vi "MNIST_Classifier_CNN(Train).vi"() -> ()   [LabVIEW 2024]
doc: "This example demonstrates the usage of Deep Learning Toolkit for solving hand written digit recognition problem with Convolutional Neural Network (CNN).\n\nDataset: MNIST http://yann.lecun.com/exdb/mnist/\nRequirements: Deep Learning Toolkit for LabVIEW."
uses:
  <vilib>/Ngene/Deep Learning Toolkit/Toolkit/NN_Train/Controls/NN_Train_Params.ctl
  <vilib>/Ngene/Deep Learning Toolkit/Toolkit/NN_Train/Controls/NN_Train_Optimizer.ctl
  <vilib>/Ngene/Deep Learning Toolkit/Toolkit/NN_Train/Controls/NN_Train_Data_Sampling.ctl
  _Controls/Img_GrayScale.ctl
  <vilib>/Ngene/Deep Learning Toolkit/Toolkit/NN_Train/Controls/NN_Train_Session_Data.ctl
  <vilib>/Ngene/Deep Learning Toolkit/Toolkit/NN_Train/Controls/NN_LR_Policy_Cfg.ctl
  <vilib>/Ngene/Deep Learning Toolkit/Toolkit/NN_Train/Controls/NN_LR_Policy_Type.ctl
  <vilib>/Ngene/Deep Learning Toolkit/Toolkit/NN_Network/Controls/NN_Device.ctl
  <vilib>/Ngene/Deep Learning Toolkit/Toolkit/NN_Layers/Layers/Conv2D/Controls/NN_Layer_Config(Conv2D).ctl
  <vilib>/Ngene/Deep Learning Toolkit/Toolkit/NN_Layers/Layers/Conv2D/Controls/NN_Layer_Params(Conv2D).ctl
  <vilib>/Ngene/Deep Learning Toolkit/Toolkit/NN_Layers/Layers/Conv2D/Controls/NN_Conv2D_Padding_Type.ctl
  <vilib>/Ngene/Deep Learning Toolkit/Toolkit/NN_Layers/Layers/BatchNorm/Controls/NN_BN_Params.ctl
  <vilib>/Ngene/Deep Learning Toolkit/Toolkit/NN_Activations/Controls/NN_Activation_Type.ctl
  <vilib>/Ngene/Deep Learning Toolkit/Toolkit/NN_Layers/Controls/NN_Layer_Init_Params.ctl
  <vilib>/Ngene/Deep Learning Toolkit/Toolkit/NN_Layers/Controls/NN_Layer_Weight_Init_Type.ctl
  <vilib>/Ngene/Deep Learning Toolkit/Toolkit/NN_Layers/Layers/FC/Controls/NN_Layer_Config(FC).ctl
  <vilib>/Ngene/Deep Learning Toolkit/Toolkit/NN_Network/Controls/NN_Save_Before_Destroy_Options.ctl
  <vilib>/Ngene/Deep Learning Toolkit/Toolkit/NN_Layers/Layers/Input/Controls/NN_Layer_Config(Input3D).ctl
  <vilib>/Ngene/Deep Learning Toolkit/Toolkit/NN_Data/API/NN_Dims(C,H,W).ctl
  <vilib>/Ngene/Deep Learning Toolkit/Toolkit/NN_Data/Controls/NN_Data_type.ctl
  <vilib>/Ngene/Deep Learning Toolkit/Toolkit/NN_Layers/Layers/Input/NN_Layer_Create(Input3D).vi
  <vilib>/Ngene/Deep Learning Toolkit/Toolkit/NN_Layers/Layers/Conv2D/NN_Layer_Create(Conv2D).vi
  <vilib>/Ngene/Deep Learning Toolkit/Toolkit/NN_Layers/Layers/FC/NN_Layer_Create(FC).vi
  <vilib>/Ngene/Deep Learning Toolkit/Toolkit/NN_Layers/Layers/SoftMax/NN_Layer_Create(SoftMax).vi
  <vilib>/Ngene/Deep Learning Toolkit/Toolkit/NN_Train/Loss_Functions/NN_Set_Loss(CrossEntropy).vi
  <vilib>/ptbypt/Filters.llb/FIR Filter PtByPt.vi
  <vilib>/Ngene/Deep Learning Toolkit/Toolkit/NN_Network/subVIs/NN_Predict/NN_Predict(In3D_Out1D).vi
  <vilib>/Ngene/Deep Learning Toolkit/Toolkit/NN_Train/Eval_Loss/NN_Eval_Test_Error_Loss/NN_Eval(In3D_Out1D).vi
  <vilib>/Ngene/Deep Learning Toolkit/Toolkit/NN_Train/Eval_Loss/NN_Calc_Cofusion_Matrix/NN_Calc_Confusion_Matrix(In3D_Out1D).vi
  <vilib>/Ngene/Deep Learning Toolkit/Toolkit/NN_Data/subVIs/Dataset_Destroy/NN_Datasets_All_Destroy(In3D_Out1D).vi
  <vilib>/Ngene/Deep Learning Toolkit/Toolkit/NN_Network/API/NN_Set_Input/3D/NN_Set_Input(3D_SGL_idx).vi
  <vilib>/Ngene/Deep Learning Toolkit/Toolkit/Deep_Learning_Toolkit_by_Ngene.lvlib
panel:
  in  "Tab":T1(tab)
  out "Train Speed (img/s)":dbl=1568.329544559763 format="%#_3p"
  out "Train Graphs":T2(graph)
  in  "Check_Vald":bool
  out "Session Data":T3={"Epochs"=0.22905263, "Tot_Iter"=102, "LR"=0.02, "LR_iter"=103}
  in  "Stop_Train":bool
  out "Train/Val_Metrics":T4={"Train_Loss"=0.05827807, "Valid_Loss"=0.04526825, "Valid_Error"=0.042666666} {"Train_Loss" format="%#_4g"; "Valid_Loss" format="%#_3g"}
  in  "LR Update Policy":T5={"Policy_Type"=enum."Step", "LR0"=0.019999999998737077, "k"=4.0, "WarmUp_Policy"=enum."Step", "WarmUp_Iter"=1, "WarmUp_Ratio"=1.0} {"WarmUp_Ratio" min=1; "WarmUp_Iter" min=1; "LR0" format="%.7f"}
  out "Train Speed (s/iter)":dbl=0.08161550003569573 format="%#_2p"
  in  "Train_Params":T7={"Optimizer"=enum."SGD", "Beta_1"=0.9, "Beta_2"=0.999, "Weight Decay(L1)"=1e-07, "Weight Decay(L2)"=1e-07, "Data_Sampling"=enum."Random"}
  out "Time_Elapsed":dbl=8.652226000092924 format="%<%H:%M:%S>t"
  out "Test_Loss":sgl=0.046575993 format="%#_3g"
  out "Test_Error":sgl=0.044
  in  "Working Dir":path=path "D:/working"
  in  "MNIST Dataset Path":path
  in  "NN_Device":T10
  out "Labels":string[](array[string])=["0", "1", "2", "3", "4", "5", "6", "7", "8", "9"]
  out "Draw Digit (280x280 px)":picture
  in  "Pen Color":u32(colorbox)=197379
  in  "Clear":bool
  out "Test Speed (img/s)":dbl=119.97888344398501 format="%#_2p"
  out "test time(s/img)":dbl=0.008334800018928945 format="%#_3p"
  out "Predictions":sgl[](array[slide])=[0.00022317072, 0.0016224136, 0.00590554, 0.9895844, 0.0010204009, 0.00023260966, 0.00083900435, 0.00020435848, 0.00020539068, 0.00016265694] scale=0.0..1.0
  in  "Pen Width":dbl=24.0
  in  "Stop Test":bool
  out "Pen Attributes":T11={"Width"=26, "Style"=enum."Solid"}
  out "image (28x28px)":sgl[][](graph)=[[-1.0, -1.0, -1.0, -1.0, -1.0, -1.0, -1.0, -1.0, -1.0, -1.0, -1.0, -1.0, -1.0, -1.0, -1.0, -1.0, -1.0, -1.0, -1.0, -1.0, -1.0, -1.0, -1.0, -1.0, -1.0, -1.0, -1.0, -1.0], [-1.0, -1.0, -1.0, -1.0, -1.0, -1.0, -1.0, -1.0, -1.0, -1.0, -1.0, -1.0, -1.0, -1.0, -1.0, -1.0, -1.0, -1.0, -1.0, -1.0, -1.0, -1.0, -1.0, -1.0, -1.0, -1.0, -1.0, -1.0], [-1.0, -1.0, -1.0, -1.0, -1.0, -1.0, -1.0, -1.0, -1.0, -1.0, -1.0, -1.0, -1.0, -1.0, -1.0, -1.0, -1.0, -1.0, -1.0, -1.0, -1.0, -1.0, -1.0, -1.0, -1.0, -1.0, -1.0, -1.0], [-1.0, -1.0, -1.0, -1.0, -1.0, -1.0, -1.0, -1.0, -1.0, -1.0, -1.0, -1.0, -1.0, -1.0, -1.0, -1.0, -1.0, -1.0, -1.0, -1.0, -1.0, -1.0, -1.0, -1.0, -1.0, -1.0, -1.0, -1.0], [-1.0, -1.0, -1.0, -1.0, -1.0, -1.0, -1.0, -1.0, -1.0, -1.0, -1.0, -1.0, -1.0, -1.0, -1.0, -1.0, -1.0, -1.0, -1.0, -1.0, -1.0, -1.0, -1.0, -1.0, -1.0, -1.0, -1.0, -1.0], [-1.0, -1.0, -1.0, -1.0, -1.0, -1.0, -1.0, -1.0, -1.0, -1.0, -1.0, -1.0, -1.0, -1.0, -1.0, -1.0, -1.0, -1.0, -1.0, -1.0, -1.0, -1.0, -1.0, -1.0, -1.0, -1.0, -1.0, -1.0], [-1.0, -1.0, -1.0, -1.0, -1.0, -1.0, -1.0, -1.0, -1.0, -1.0, -1.0, -1.0, -1.0, -1.0, -1.0, -1.0, -1.0, -1.0, -1.0, -1.0, -1.0, -1.0, -1.0, -1.0, -1.0, -1.0, -1.0, -1.0], [-1.0, -1.0, -1.0, -1.0, -1.0, -1.0, -1.0, -1.0, -1.0, -1.0, -1.0, -1.0, -1.0, -1.0, -1.0, -1.0, -1.0, -1.0, -1.0, -1.0, -1.0, -1.0, -1.0, -1.0, -1.0, -1.0, -1.0, -1.0], [-1.0, -1.0, -1.0, -1.0, -1.0, -1.0, -1.0, -1.0, -1.0, -1.0, -1.0, -1.0, -1.0, -1.0, -1.0, -1.0, -1.0, -1.0, -1.0, -1.0, -1.0, -1.0, -1.0, -1.0, -1.0, -1.0, -1.0, -1.0], [-1.0, -1.0, -1.0, -1.0, -1.0, -1.0, -1.0, -1.0, -1.0, -1.0, -1.0, -1.0, -1.0, -1.0, -1.0, -1.0, -1.0, -1.0, -1.0, -1.0, -1.0, -1.0, -1.0, -1.0, -1.0, -1.0, -1.0, -1.0], [-1.0, -1.0, -1.0, -1.0, -1.0, -1.0, -1.0, -1.0, -1.0, -1.0, -1.0, -1.0, -1.0, -1.0, -1.0, -1.0, -1.0, -1.0, -1.0, -1.0, -1.0, -1.0, -1.0, -1.0, -1.0, -1.0, -1.0, -1.0], [-1.0, -1.0, -1.0, -1.0, -1.0, -1.0, -1.0, -1.0, -1.0, -1.0, -1.0, -1.0, -1.0, -1.0, -1.0, -1.0, -1.0, -1.0, -1.0, -1.0, -1.0, -1.0, -1.0, -1.0, -1.0, -1.0, -1.0, -1.0], [-1.0, -1.0, -1.0, -1.0, -1.0, -1.0, -1.0, -1.0, -1.0, -1.0, -1.0, -1.0, -1.0, -1.0, -1.0, -1.0, -1.0, -1.0, -1.0, -1.0, -1.0, -1.0, -1.0, -1.0, -1.0, -1.0, -1.0, -1.0], [-1.0, -1.0, -1.0, -1.0, -1.0, -1.0, -1.0, -1.0, -1.0, -1.0, -1.0, -1.0, -1.0, -1.0, -1.0, -1.0, -1.0, -1.0, -1.0, -1.0, -1.0, -1.0, -1.0, -1.0, -1.0, -1.0, -1.0, -1.0], [-1.0, -1.0, -1.0, -1.0, -1.0, -1.0, -1.0, -1.0, -1.0, -1.0, -1.0, -1.0, -1.0, -1.0, -1.0, -1.0, -1.0, -1.0, -1.0, -1.0, -1.0, -1.0, -1.0, -1.0, -1.0, -1.0, -1.0, -1.0], [-1.0, -1.0, -1.0, -1.0, -1.0, -1.0, -1.0, -1.0, -1.0, -1.0, -1.0, -1.0, -1.0, -1.0, -1.0, -1.0, -1.0, -1.0, -1.0, -1.0, -1.0, -1.0, -1.0, -1.0, -1.0, -1.0, -1.0, -1.0], [-1.0, -1.0, -1.0, -1.0, -1.0, -1.0, -1.0, -1.0, -1.0, -1.0, -1.0, -1.0, -1.0, -1.0, -1.0, -1.0, -1.0, -1.0, -1.0, -1.0, -1.0, -1.0, -1.0, -1.0, -1.0, -1.0, -1.0, -1.0], [-1.0, -1.0, -1.0, -1.0, -1.0, -1.0, -1.0, -1.0, -1.0, -1.0, -1.0, -1.0, -1.0, -1.0, -1.0, -1.0, -1.0, -1.0, -1.0, -1.0, -1.0, -1.0, -1.0, -1.0, -1.0, -1.0, -1.0, -1.0], [-1.0, -1.0, -1.0, -1.0, -1.0, -1.0, -1.0, -1.0, -1.0, -1.0, -1.0, -1.0, -1.0, -1.0, -1.0, -1.0, -1.0, -1.0, -1.0, -1.0, -1.0, -1.0, -1.0, -1.0, -1.0, -1.0, -1.0, -1.0], [-1.0, -1.0, -1.0, -1.0, -1.0, -1.0, -1.0, -1.0, -1.0, -1.0, -1.0, -1.0, -1.0, -1.0, -1.0, -1.0, -1.0, -1.0, -1.0, -1.0, -1.0, -1.0, -1.0, -1.0, -1.0, -1.0, -1.0, -1.0], [-1.0, -1.0, -1.0, -1.0, -1.0, -1.0, -1.0, -1.0, -1.0, -1.0, -1.0, -1.0, -1.0, -1.0, -1.0, -1.0, -1.0, -1.0, -1.0, -1.0, -1.0, -1.0, -1.0, -1.0, -1.0, -1.0, -1.0, -1.0], [-1.0, -1.0, -1.0, -1.0, -1.0, -1.0, -1.0, -1.0, -1.0, -1.0, -1.0, -1.0, -1.0, -1.0, -1.0, -1.0, -1.0, -1.0, -1.0, -1.0, -1.0, -1.0, -1.0, -1.0, -1.0, -1.0, -1.0, -1.0], [-1.0, -1.0, -1.0, -1.0, -1.0, -1.0, -1.0, -1.0, -1.0, -1.0, -1.0, -1.0, -1.0, -1.0, -1.0, -1.0, -1.0, -1.0, -1.0, -1.0, -1.0, -1.0, -1.0, -1.0, -1.0, -1.0, -1.0, -1.0], [-1.0, -1.0, -1.0, -1.0, -1.0, -1.0, -1.0, -1.0, -1.0, -1.0, -1.0, -1.0, -1.0, -1.0, -1.0, -1.0, -1.0, -1.0, -1.0, -1.0, -1.0, -1.0, -1.0, -1.0, -1.0, -1.0, -1.0, -1.0], [-1.0, -1.0, -1.0, -1.0, -1.0, -1.0, -1.0, -1.0, -1.0, -1.0, -1.0, -1.0, -1.0, -1.0, -1.0, -1.0, -1.0, -1.0, -1.0, -1.0, -1.0, -1.0, -1.0, -1.0, -1.0, -1.0, -1.0, -1.0], [-1.0, -1.0, -1.0, -1.0, -1.0, -1.0, -1.0, -1.0, -1.0, -1.0, -1.0, -1.0, -1.0, -1.0, -1.0, -1.0, -1.0, -1.0, -1.0, -1.0, -1.0, -1.0, -1.0, -1.0, -1.0, -1.0, -1.0, -1.0], [-1.0, -1.0, -1.0, -1.0, -1.0, -1.0, -1.0, -1.0, -1.0, -1.0, -1.0, -1.0, -1.0, -1.0, -1.0, -1.0, -1.0, -1.0, -1.0, -1.0, -1.0, -1.0, -1.0, -1.0, -1.0, -1.0, -1.0, -1.0], [-1.0, -1.0, -1.0, -1.0, -1.0, -1.0, -1.0, -1.0, -1.0, -1.0, -1.0, -1.0, -1.0, -1.0, -1.0, -1.0, -1.0, -1.0, -1.0, -1.0, -1.0, -1.0, -1.0, -1.0, -1.0, -1.0, -1.0, -1.0]]
  out "Incorrectly Classified Imgs":T12[][](array[typedef])=[[{"image"=array28x28[784 elements], "Truth"=2, "Predicted"=2}, {"image"=array28x28[784 elements], "Truth"=9, "Predicted"=9}, {"image"=array28x28[784 elements], "Truth"=2, "Predicted"=2}, {"image"=array28x28[784 elements], "Truth"=7, "Predicted"=7}, {"image"=array28x28[784 elements], "Truth"=8, "Predicted"=8}, {"image"=array28x28[784 elements], "Truth"=2, "Predicted"=2}, {"image"=array28x28[784 elements], "Truth"=0, "Predicted"=0}, {"image"=array28x28[784 elements], "Truth"=1, "Predicted"=1}, {"image"=array28x28[784 elements], "Truth"=7, "Predicted"=7}, {"image"=array28x28[784 elements], "Truth"=3, "Predicted"=3}], [{"image"=array28x28[784 elements], "Truth"=7, "Predicted"=7}, {"image"=array28x28[784 elements], "Truth"=7, "Predicted"=7}, {"image"=array28x28[784 elements], "Truth"=7, "Predicted"=7}, {"image"=array28x28[784 elements], "Truth"=7, "Predicted"=7}, {"image"=array28x28[784 elements], "Truth"=0, "Predicted"=0}, {"image"=array28x28[784 elements], "Truth"=5, "Predicted"=5}, {"image"=array28x28[784 elements], "Truth"=2, "Predicted"=2}, {"image"=array28x28[784 elements], "Truth"=5, "Predicted"=5}, {"image"=array28x28[784 elements], "Truth"=8, "Predicted"=8}, {"image"=array28x28[784 elements], "Truth"=5, "Predicted"=5}], [{"image"=array28x28[784 elements], "Truth"=1, "Predicted"=1}, {"image"=array28x28[784 elements], "Truth"=9, "Predicted"=9}, {"image"=array28x28[784 elements], "Truth"=7, "Predicted"=7}, {"image"=array28x28[784 elements], "Truth"=2, "Predicted"=2}, {"image"=array28x28[784 elements], "Truth"=3, "Predicted"=3}, {"image"=array28x28[784 elements], "Truth"=9, "Predicted"=9}, {"image"=array28x28[784 elements], "Truth"=2, "Predicted"=2}, {"image"=array28x28[784 elements], "Truth"=7, "Predicted"=7}, {"image"=array28x28[784 elements], "Truth"=8, "Predicted"=8}, {"image"=array28x28[784 elements], "Truth"=4, "Predicted"=4}], [{"image"=array28x28[784 elements], "Truth"=0, "Predicted"=0}, {"image"=array28x28[784 elements], "Truth"=8, "Predicted"=8}, {"image"=array28x28[784 elements], "Truth"=3, "Predicted"=3}, {"image"=array28x28[784 elements], "Truth"=4, "Predicted"=4}, {"image"=array28x28[784 elements], "Truth"=9, "Predicted"=9}, {"image"=array28x28[784 elements], "Truth"=6, "Predicted"=6}, {"image"=array28x28[784 elements], "Truth"=9, "Predicted"=9}, {"image"=array28x28[784 elements], "Truth"=9, "Predicted"=9}, {"image"=array28x28[784 elements], "Truth"=5, "Predicted"=5}, {"image"=array28x28[784 elements], "Truth"=9, "Predicted"=9}], [{"image"=array28x28[784 elements], "Truth"=3, "Predicted"=3}, {"image"=array28x28[784 elements], "Truth"=7, "Predicted"=7}, {"image"=array28x28[784 elements], "Truth"=9, "Predicted"=9}, {"image"=array28x28[784 elements], "Truth"=7, "Predicted"=7}, {"image"=array28x28[784 elements], "Truth"=3, "Predicted"=3}, {"image"=array28x28[784 elements], "Truth"=7, "Predicted"=7}, {"image"=array28x28[784 elements], "Truth"=5, "Predicted"=5}, {"image"=array28x28[784 elements], "Truth"=7, "Predicted"=7}, {"image"=array28x28[784 elements], "Truth"=6, "Predicted"=6}, {"image"=array28x28[784 elements], "Truth"=9, "Predicted"=9}], [{"image"=array28x28[784 elements], "Truth"=0, "Predicted"=0}, {"image"=array28x28[784 elements], "Truth"=9, "Predicted"=9}, {"image"=array28x28[784 elements], "Truth"=2, "Predicted"=2}, {"image"=array28x28[784 elements], "Truth"=9, "Predicted"=9}, {"image"=array28x28[784 elements], "Truth"=5, "Predicted"=5}, {"image"=array28x28[784 elements], "Truth"=1, "Predicted"=1}, {"image"=array28x28[784 elements], "Truth"=8, "Predicted"=8}, {"image"=array28x28[784 elements], "Truth"=7, "Predicted"=7}, {"image"=array28x28[784 elements], "Truth"=4, "Predicted"=4}, {"image"=array28x28[784 elements], "Truth"=0, "Predicted"=0}], [{"image"=array28x28[784 elements], "Truth"=8, "Predicted"=8}, {"image"=array28x28[784 elements], "Truth"=6, "Predicted"=6}, {"image"=array28x28[784 elements], "Truth"=8, "Predicted"=8}, {"image"=array28x28[784 elements], "Truth"=1, "Predicted"=1}, {"image"=array28x28[784 elements], "Truth"=7, "Predicted"=7}, {"image"=array28x28[784 elements], "Truth"=7, "Predicted"=7}, {"image"=array28x28[784 elements], "Truth"=7, "Predicted"=7}, {"image"=array28x28[784 elements], "Truth"=2, "Predicted"=2}, {"image"=array28x28[784 elements], "Truth"=2, "Predicted"=2}, {"image"=array28x28[784 elements], "Truth"=4, "Predicted"=4}], [{"image"=array28x28[784 elements], "Truth"=5, "Predicted"=5}, {"image"=array28x28[784 elements], "Truth"=6, "Predicted"=6}, {"image"=array28x28[784 elements], "Truth"=1, "Predicted"=1}, {"image"=array28x28[784 elements], "Truth"=9, "Predicted"=9}, {"image"=array28x28[784 elements], "Truth"=9, "Predicted"=9}, {"image"=array28x28[784 elements], "Truth"=7, "Predicted"=7}, {"image"=array28x28[784 elements], "Truth"=3, "Predicted"=3}, {"image"=array28x28[784 elements], "Truth"=2, "Predicted"=2}, {"image"=array28x28[784 elements], "Truth"=6, "Predicted"=6}, {"image"=array28x28[784 elements], "Truth"=3, "Predicted"=3}], [{"image"=array28x28[784 elements], "Truth"=9, "Predicted"=9}, {"image"=array28x28[784 elements], "Truth"=5, "Predicted"=5}, {"image"=array28x28[784 elements], "Truth"=1, "Predicted"=1}, {"image"=array28x28[784 elements], "Truth"=0, "Predicted"=0}, {"image"=array28x28[784 elements], "Truth"=5, "Predicted"=5}, {"image"=array28x28[784 elements], "Truth"=7, "Predicted"=7}, {"image"=array28x28[784 elements], "Truth"=2, "Predicted"=2}, {"image"=array28x28[784 elements], "Truth"=5, "Predicted"=5}, {"image"=array28x28[784 elements], "Truth"=7, "Predicted"=7}, {"image"=array28x28[784 elements], "Truth"=4, "Predicted"=4}], [{"image"=array28x28[784 elements], "Truth"=9, "Predicted"=9}, {"image"=array28x28[784 elements], "Truth"=9, "Predicted"=9}, {"image"=array28x28[784 elements], "Truth"=5, "Predicted"=5}, {"image"=array28x28[784 elements], "Truth"=5, "Predicted"=5}, {"image"=array28x28[784 elements], "Truth"=3, "Predicted"=3}, {"image"=array28x28[784 elements], "Truth"=6, "Predicted"=6}, {"image"=array28x28[784 elements], "Truth"=7, "Predicted"=7}, {"image"=array28x28[784 elements], "Truth"=7, "Predicted"=7}, {"image"=array28x28[784 elements], "Truth"=7, "Predicted"=7}, {"image"=array28x28[784 elements], "Truth"=3, "Predicted"=3}], [{"image"=array28x28[784 elements], "Truth"=3, "Predicted"=3}, {"image"=array28x28[784 elements], "Truth"=7, "Predicted"=7}, {"image"=array28x28[784 elements], "Truth"=5, "Predicted"=5}, {"image"=array28x28[784 elements], "Truth"=3, "Predicted"=3}, {"image"=array28x28[784 elements], "Truth"=2, "Predicted"=2}, {"image"=array28x28[784 elements], "Truth"=5, "Predicted"=5}, {"image"=array28x28[784 elements], "Truth"=7, "Predicted"=7}, {"image"=array28x28[784 elements], "Truth"=9, "Predicted"=9}, {"image"=array28x28[784 elements], "Truth"=4, "Predicted"=4}, {"image"=array28x28[784 elements], "Truth"=5, "Predicted"=5}], [{"image"=array28x28[784 elements], "Truth"=9, "Predicted"=9}, {"image"=array28x28[784 elements], "Truth"=7, "Predicted"=7}, {"image"=array28x28[784 elements], "Truth"=5, "Predicted"=5}, {"image"=array28x28[784 elements], "Truth"=3, "Predicted"=3}, {"image"=array28x28[784 elements], "Truth"=0, "Predicted"=0}, {"image"=array28x28[784 elements], "Truth"=9, "Predicted"=9}, {"image"=array28x28[784 elements], "Truth"=4, "Predicted"=4}, {"image"=array28x28[784 elements], "Truth"=3, "Predicted"=3}, {"image"=array28x28[784 elements], "Truth"=4, "Predicted"=4}, {"image"=array28x28[784 elements], "Truth"=6, "Predicted"=6}], [{"image"=array28x28[784 elements], "Truth"=5, "Predicted"=5}, {"image"=array28x28[784 elements], "Truth"=5, "Predicted"=5}, {"image"=array28x28[784 elements], "Truth"=0, "Predicted"=0}, {"image"=array28x28[784 elements], "Truth"=9, "Predicted"=9}, {"image"=array28x28[784 elements], "Truth"=2, "Predicted"=2}, {"image"=array28x28[784 elements], "Truth"=3, "Predicted"=3}, {"image"=array28x28[784 elements], "Truth"=8, "Predicted"=8}, {"image"=array28x28[784 elements], "Truth"=7, "Predicted"=7}, {"image"=array28x28[784 elements], "Truth"=9, "Predicted"=9}, {"image"=array28x28[784 elements], "Truth"=9, "Predicted"=9}], [{"image"=array28x28[784 elements], "Truth"=0, "Predicted"=0}, {"image"=array28x28[784 elements], "Truth"=9, "Predicted"=9}, {"image"=array28x28[784 elements], "Truth"=7, "Predicted"=7}, {"image"=array28x28[784 elements], "Truth"=0, "Predicted"=0}, {"image"=array28x28[784 elements], "Truth"=2, "Predicted"=2}, {"image"=array28x28[784 elements], "Truth"=9, "Predicted"=9}, {"image"=array28x28[784 elements], "Truth"=1, "Predicted"=1}, {"image"=array28x28[784 elements], "Truth"=9, "Predicted"=9}, {"image"=array28x28[784 elements], "Truth"=5, "Predicted"=5}, {"image"=array28x28[784 elements], "Truth"=2, "Predicted"=2}], [{"image"=array28x28[784 elements], "Truth"=8, "Predicted"=8}, {"image"=array28x28[784 elements], "Truth"=5, "Predicted"=5}, {"image"=array28x28[784 elements], "Truth"=1, "Predicted"=1}, {"image"=array28x28[784 elements], "Truth"=6, "Predicted"=6}, {"image"=array28x28[784 elements], "Truth"=9, "Predicted"=9}, {"image"=array28x28[784 elements], "Truth"=6, "Predicted"=6}, {"image"=array28x28[784 elements], "Truth"=0, "Predicted"=0}, {"image"=array28x28[784 elements], "Truth"=7, "Predicted"=7}, {"image"=array28x28[784 elements], "Truth"=9, "Predicted"=9}, {"image"=array28x28[784 elements], "Truth"=9, "Predicted"=9}], [{"image"=array28x28[784 elements], "Truth"=7, "Predicted"=7}, {"image"=array28x28[784 elements], "Truth"=1, "Predicted"=1}, {"image"=array28x28[784 elements], "Truth"=5, "Predicted"=5}, {"image"=array28x28[784 elements], "Truth"=9, "Predicted"=9}, {"image"=array28x28[784 elements], "Truth"=3, "Predicted"=3}, {"image"=array28x28[784 elements], "Truth"=9, "Predicted"=9}, {"image"=array28x28[784 elements], "Truth"=4, "Predicted"=4}, {"image"=array28x28[784 elements], "Truth"=9, "Predicted"=9}, {"image"=array28x28[784 elements], "Truth"=9, "Predicted"=9}, {"image"=array28x28[784 elements], "Truth"=6, "Predicted"=6}], [{"image"=array28x28[784 elements], "Truth"=9, "Predicted"=9}, {"image"=array28x28[784 elements], "Truth"=2, "Predicted"=2}, {"image"=array28x28[784 elements], "Truth"=8, "Predicted"=8}, {"image"=array28x28[784 elements], "Truth"=8, "Predicted"=8}, {"image"=array28x28[784 elements], "Truth"=5, "Predicted"=5}, {"image"=array28x28[784 elements], "Truth"=1, "Predicted"=1}, {"image"=array28x28[784 elements], "Truth"=7, "Predicted"=7}, {"image"=array28x28[784 elements], "Truth"=0, "Predicted"=0}, {"image"=array28x28[784 elements], "Truth"=5, "Predicted"=5}, {"image"=array28x28[784 elements], "Truth"=9, "Predicted"=9}], [{"image"=array28x28[784 elements], "Truth"=5, "Predicted"=5}, {"image"=array28x28[784 elements], "Truth"=3, "Predicted"=3}, {"image"=array28x28[784 elements], "Truth"=0, "Predicted"=0}, {"image"=array28x28[784 elements], "Truth"=9, "Predicted"=9}, {"image"=array28x28[784 elements], "Truth"=2, "Predicted"=2}, {"image"=array28x28[784 elements], "Truth"=2, "Predicted"=2}, {"image"=array28x28[784 elements], "Truth"=5, "Predicted"=5}, {"image"=array28x28[784 elements], "Truth"=5, "Predicted"=5}, {"image"=array28x28[784 elements], "Truth"=3, "Predicted"=3}, {"image"=array28x28[784 elements], "Truth"=7, "Predicted"=7}], [{"image"=array28x28[784 elements], "Truth"=9, "Predicted"=9}, {"image"=array28x28[784 elements], "Truth"=9, "Predicted"=9}, {"image"=array28x28[784 elements], "Truth"=7, "Predicted"=7}, {"image"=array28x28[784 elements], "Truth"=8, "Predicted"=8}, {"image"=array28x28[784 elements], "Truth"=7, "Predicted"=7}, {"image"=array28x28[784 elements], "Truth"=3, "Predicted"=3}, {"image"=array28x28[784 elements], "Truth"=3, "Predicted"=3}, {"image"=array28x28[784 elements], "Truth"=6, "Predicted"=6}, {"image"=array28x28[784 elements], "Truth"=9, "Predicted"=9}, {"image"=array28x28[784 elements], "Truth"=0, "Predicted"=0}], [{"image"=array28x28[784 elements], "Truth"=2, "Predicted"=2}, {"image"=array28x28[784 elements], "Truth"=9, "Predicted"=9}, {"image"=array28x28[784 elements], "Truth"=9, "Predicted"=9}, {"image"=array28x28[784 elements], "Truth"=2, "Predicted"=2}, {"image"=array28x28[784 elements], "Truth"=0, "Predicted"=0}, {"image"=array28x28[784 elements], "Truth"=7, "Predicted"=7}, {"image"=array28x28[784 elements], "Truth"=9, "Predicted"=9}, {"image"=array28x28[784 elements], "Truth"=9, "Predicted"=9}, {"image"=array28x28[784 elements], "Truth"=7, "Predicted"=7}, {"image"=array28x28[784 elements], "Truth"=9, "Predicted"=9}], [{"image"=array28x28[784 elements], "Truth"=9, "Predicted"=9}, {"image"=array28x28[784 elements], "Truth"=9, "Predicted"=9}, {"image"=array28x28[784 elements], "Truth"=0, "Predicted"=0}, {"image"=array28x28[784 elements], "Truth"=9, "Predicted"=9}, {"image"=array28x28[784 elements], "Truth"=7, "Predicted"=7}, {"image"=array28x28[784 elements], "Truth"=9, "Predicted"=9}, {"image"=array28x28[784 elements], "Truth"=1, "Predicted"=1}, {"image"=array28x28[784 elements], "Truth"=7, "Predicted"=7}, {"image"=array28x28[784 elements], "Truth"=4, "Predicted"=4}, {"image"=array28x28[784 elements], "Truth"=2, "Predicted"=2}], [{"image"=array28x28[784 elements], "Truth"=5, "Predicted"=5}, {"image"=array28x28[784 elements], "Truth"=0, "Predicted"=0}, {"image"=array28x28[784 elements], "Truth"=5, "Predicted"=5}, {"image"=array28x28[784 elements], "Truth"=7, "Predicted"=7}, {"image"=array28x28[784 elements], "Truth"=3, "Predicted"=3}, {"image"=array28x28[784 elements], "Truth"=3, "Predicted"=3}, {"image"=array28x28[784 elements], "Truth"=3, "Predicted"=3}, {"image"=array28x28[784 elements], "Truth"=3, "Predicted"=3}, {"image"=array28x28[784 elements], "Truth"=9, "Predicted"=9}, {"image"=array28x28[784 elements], "Truth"=9, "Predicted"=9}], [{"image"=array28x28[784 elements], "Truth"=5, "Predicted"=5}, {"image"=array28x28[784 elements], "Truth"=2, "Predicted"=2}, {"image"=array28x28[784 elements], "Truth"=6, "Predicted"=6}, {"image"=array28x28[784 elements], "Truth"=8, "Predicted"=8}, {"image"=array28x28[784 elements], "Truth"=7, "Predicted"=7}, {"image"=array28x28[784 elements], "Truth"=1, "Predicted"=1}, {"image"=array28x28[784 elements], "Truth"=3, "Predicted"=3}, {"image"=array28x28[784 elements], "Truth"=6, "Predicted"=6}, {"image"=array28x28[784 elements], "Truth"=7, "Predicted"=7}, {"image"=array28x28[784 elements], "Truth"=1, "Predicted"=1}], [{"image"=array28x28[784 elements], "Truth"=0, "Predicted"=0}, {"image"=array28x28[784 elements], "Truth"=4, "Predicted"=4}, {"image"=array28x28[784 elements], "Truth"=3, "Predicted"=3}, {"image"=array28x28[784 elements], "Truth"=3, "Predicted"=3}, {"image"=array28x28[784 elements], "Truth"=6, "Predicted"=6}, {"image"=array28x28[784 elements], "Truth"=5, "Predicted"=5}, {"image"=array28x28[784 elements], "Truth"=1, "Predicted"=1}, {"image"=array28x28[784 elements], "Truth"=7, "Predicted"=7}, {"image"=array28x28[784 elements], "Truth"=9, "Predicted"=9}, {"image"=array28x28[784 elements], "Truth"=1, "Predicted"=1}], [{"image"=array28x28[784 elements], "Truth"=5, "Predicted"=5}, {"image"=array28x28[784 elements], "Truth"=9, "Predicted"=9}, {"image"=array28x28[784 elements], "Truth"=6, "Predicted"=6}, {"image"=array28x28[784 elements], "Truth"=0, "Predicted"=0}, {"image"=array28x28[784 elements], "Truth"=3, "Predicted"=3}, {"image"=array28x28[784 elements], "Truth"=3, "Predicted"=3}, {"image"=array28x28[784 elements], "Truth"=2, "Predicted"=2}, {"image"=array28x28[784 elements], "Truth"=1, "Predicted"=1}, {"image"=array28x28[784 elements], "Truth"=0, "Predicted"=0}, {"image"=array28x28[784 elements], "Truth"=7, "Predicted"=7}], [{"image"=array28x28[784 elements], "Truth"=5, "Predicted"=5}, {"image"=array28x28[784 elements], "Truth"=6, "Predicted"=6}, {"image"=array28x28[784 elements], "Truth"=5, "Predicted"=5}, {"image"=array28x28[784 elements], "Truth"=3, "Predicted"=3}, {"image"=array28x28[784 elements], "Truth"=7, "Predicted"=7}, {"image"=array28x28[784 elements], "Truth"=9, "Predicted"=9}, {"image"=array28x28[784 elements], "Truth"=0, "Predicted"=0}, {"image"=array28x28[784 elements], "Truth"=7, "Predicted"=7}, {"image"=array28x28[784 elements], "Truth"=6, "Predicted"=6}, {"image"=array28x28[784 elements], "Truth"=7, "Predicted"=7}], [{"image"=array28x28[784 elements], "Truth"=9, "Predicted"=9}, {"image"=array28x28[784 elements], "Truth"=6, "Predicted"=6}, {"image"=array28x28[784 elements], "Truth"=9, "Predicted"=9}, {"image"=array28x28[784 elements], "Truth"=4, "Predicted"=4}, {"image"=array28x28[784 elements], "Truth"=3, "Predicted"=3}, {"image"=array28x28[784 elements], "Truth"=7, "Predicted"=7}, {"image"=array28x28[784 elements], "Truth"=2, "Predicted"=2}, {"image"=array28x28[784 elements], "Truth"=2, "Predicted"=2}, {"image"=array28x28[784 elements], "Truth"=0, "Predicted"=0}, {"image"=array28x28[784 elements], "Truth"=7, "Predicted"=7}], [{"image"=array28x28[784 elements], "Truth"=7, "Predicted"=7}, {"image"=array28x28[784 elements], "Truth"=3, "Predicted"=3}, {"image"=array28x28[784 elements], "Truth"=1, "Predicted"=1}, {"image"=array28x28[784 elements], "Truth"=7, "Predicted"=7}, {"image"=array28x28[784 elements], "Truth"=5, "Predicted"=5}, {"image"=array28x28[784 elements], "Truth"=4, "Predicted"=4}, {"image"=array28x28[784 elements], "Truth"=9, "Predicted"=9}, {"image"=array28x28[784 elements], "Truth"=2, "Predicted"=2}, {"image"=array28x28[784 elements], "Truth"=9, "Predicted"=9}, {"image"=array28x28[784 elements], "Truth"=4, "Predicted"=4}], [{"image"=array28x28[784 elements], "Truth"=9, "Predicted"=9}, {"image"=array28x28[784 elements], "Truth"=3, "Predicted"=3}, {"image"=array28x28[784 elements], "Truth"=2, "Predicted"=2}, {"image"=array28x28[784 elements], "Truth"=7, "Predicted"=7}, {"image"=array28x28[784 elements], "Truth"=7, "Predicted"=7}, {"image"=array28x28[784 elements], "Truth"=4, "Predicted"=4}, {"image"=array28x28[784 elements], "Truth"=8, "Predicted"=8}, {"image"=array28x28[784 elements], "Truth"=0, "Predicted"=0}, {"image"=array28x28[784 elements], "Truth"=0, "Predicted"=0}, {"image"=array28x28[784 elements], "Truth"=4, "Predicted"=4}], [{"image"=array28x28[784 elements], "Truth"=2, "Predicted"=2}, {"image"=array28x28[784 elements], "Truth"=9, "Predicted"=9}, {"image"=array28x28[784 elements], "Truth"=0, "Predicted"=0}, {"image"=array28x28[784 elements], "Truth"=6, "Predicted"=6}, {"image"=array28x28[784 elements], "Truth"=5, "Predicted"=5}, {"image"=array28x28[784 elements], "Truth"=1, "Predicted"=1}, {"image"=array28x28[784 elements], "Truth"=5, "Predicted"=5}, {"image"=array28x28[784 elements], "Truth"=4, "Predicted"=4}, {"image"=array28x28[784 elements], "Truth"=7, "Predicted"=7}, {"image"=array28x28[784 elements], "Truth"=3, "Predicted"=3}], [{"image"=array28x28[784 elements], "Truth"=4, "Predicted"=4}, {"image"=array28x28[784 elements], "Truth"=1, "Predicted"=1}, {"image"=array28x28[784 elements], "Truth"=7, "Predicted"=7}, {"image"=array28x28[784 elements], "Truth"=2, "Predicted"=2}, {"image"=array28x28[784 elements], "Truth"=4, "Predicted"=4}, {"image"=array28x28[784 elements], "Truth"=9, "Predicted"=9}, {"image"=array28x28[784 elements], "Truth"=8, "Predicted"=8}, {"image"=array28x28[784 elements], "Truth"=3, "Predicted"=3}, {"image"=array28x28[784 elements], "Truth"=9, "Predicted"=9}, {"image"=array28x28[784 elements], "Truth"=9, "Predicted"=9}], [{"image"=array28x28[784 elements], "Truth"=4, "Predicted"=4}, {"image"=array28x28[784 elements], "Truth"=6, "Predicted"=6}, {"image"=array28x28[784 elements], "Truth"=9, "Predicted"=9}, {"image"=array28x28[784 elements], "Truth"=3, "Predicted"=3}, {"image"=array28x28[784 elements], "Truth"=5, "Predicted"=5}, {"image"=array28x28[784 elements], "Truth"=1, "Predicted"=1}, {"image"=array28x28[784 elements], "Truth"=5, "Predicted"=5}, {"image"=array28x28[784 elements], "Truth"=7, "Predicted"=7}, {"image"=array28x28[784 elements], "Truth"=5, "Predicted"=5}, {"image"=array28x28[784 elements], "Truth"=7, "Predicted"=7}], [{"image"=array28x28[784 elements], "Truth"=9, "Predicted"=9}, {"image"=array28x28[784 elements], "Truth"=0, "Predicted"=0}, {"image"=array28x28[784 elements], "Truth"=0, "Predicted"=0}, {"image"=array28x28[784 elements], "Truth"=3, "Predicted"=3}, {"image"=array28x28[784 elements], "Truth"=9, "Predicted"=9}, {"image"=array28x28[784 elements], "Truth"=8, "Predicted"=8}, {"image"=array28x28[784 elements], "Truth"=9, "Predicted"=9}, {"image"=array28x28[784 elements], "Truth"=5, "Predicted"=5}, {"image"=array28x28[784 elements], "Truth"=9, "Predicted"=9}, {"image"=array28x28[784 elements], "Truth"=9, "Predicted"=9}], [{"image"=array28x28[784 elements], "Truth"=5, "Predicted"=5}, {"image"=array28x28[784 elements], "Truth"=5, "Predicted"=5}, {"image"=array28x28[784 elements], "Truth"=5, "Predicted"=5}, {"image"=array28x28[784 elements], "Truth"=5, "Predicted"=5}, {"image"=array28x28[784 elements], "Truth"=5, "Predicted"=5}, {"image"=array28x28[784 elements], "Truth"=2, "Predicted"=2}, {"image"=array28x28[784 elements], "Truth"=6, "Predicted"=6}, {"image"=array28x28[784 elements], "Truth"=0, "Predicted"=0}, {"image"=array28x28[784 elements], "Truth"=7, "Predicted"=7}, {"image"=array28x28[784 elements], "Truth"=5, "Predicted"=5}], [{"image"=array28x28[784 elements], "Truth"=7, "Predicted"=7}, {"image"=array28x28[784 elements], "Truth"=7, "Predicted"=7}, {"image"=array28x28[784 elements], "Truth"=7, "Predicted"=7}, {"image"=array28x28[784 elements], "Truth"=5, "Predicted"=5}, {"image"=array28x28[784 elements], "Truth"=7, "Predicted"=7}, {"image"=array28x28[784 elements], "Truth"=5, "Predicted"=5}, {"image"=array28x28[784 elements], "Truth"=5, "Predicted"=5}, {"image"=array28x28[784 elements], "Truth"=9, "Predicted"=9}, {"image"=array28x28[784 elements], "Truth"=5, "Predicted"=5}, {"image"=array28x28[784 elements], "Truth"=9, "Predicted"=9}], [{"image"=array28x28[784 elements], "Truth"=4, "Predicted"=4}, {"image"=array28x28[784 elements], "Truth"=9, "Predicted"=9}, {"image"=array28x28[784 elements], "Truth"=7, "Predicted"=7}, {"image"=array28x28[784 elements], "Truth"=7, "Predicted"=7}, {"image"=array28x28[784 elements], "Truth"=7, "Predicted"=7}, {"image"=array28x28[784 elements], "Truth"=5, "Predicted"=5}, {"image"=array28x28[784 elements], "Truth"=7, "Predicted"=7}, {"image"=array28x28[784 elements], "Truth"=0, "Predicted"=0}, {"image"=array28x28[784 elements], "Truth"=2, "Predicted"=2}, {"image"=array28x28[784 elements], "Truth"=8, "Predicted"=8}], [{"image"=array28x28[784 elements], "Truth"=5, "Predicted"=5}, {"image"=array28x28[784 elements], "Truth"=7, "Predicted"=7}, {"image"=array28x28[784 elements], "Truth"=7, "Predicted"=7}, {"image"=array28x28[784 elements], "Truth"=3, "Predicted"=3}, {"image"=array28x28[784 elements], "Truth"=9, "Predicted"=9}, {"image"=array28x28[784 elements], "Truth"=9, "Predicted"=9}, {"image"=array28x28[784 elements], "Truth"=8, "Predicted"=8}, {"image"=array28x28[784 elements], "Truth"=8, "Predicted"=8}, {"image"=array28x28[784 elements], "Truth"=8, "Predicted"=8}, {"image"=array28x28[784 elements], "Truth"=2, "Predicted"=2}], [{"image"=array28x28[784 elements], "Truth"=2, "Predicted"=2}, {"image"=array28x28[784 elements], "Truth"=8, "Predicted"=8}, {"image"=array28x28[784 elements], "Truth"=9, "Predicted"=9}, {"image"=array28x28[784 elements], "Truth"=8, "Predicted"=8}, {"image"=array28x28[784 elements], "Truth"=6, "Predicted"=6}, {"image"=array28x28[784 elements], "Truth"=8, "Predicted"=8}, {"image"=array28x28[784 elements], "Truth"=8, "Predicted"=8}, {"image"=array28x28[784 elements], "Truth"=9, "Predicted"=9}, {"image"=array28x28[784 elements], "Truth"=5, "Predicted"=5}, {"image"=array28x28[784 elements], "Truth"=9, "Predicted"=9}], [{"image"=array28x28[784 elements], "Truth"=5, "Predicted"=5}, {"image"=array28x28[784 elements], "Truth"=5, "Predicted"=5}, {"image"=array28x28[784 elements], "Truth"=7, "Predicted"=7}, {"image"=array28x28[784 elements], "Truth"=4, "Predicted"=4}, {"image"=array28x28[784 elements], "Truth"=6, "Predicted"=6}, {"image"=array28x28[784 elements], "Truth"=9, "Predicted"=9}, {"image"=array28x28[784 elements], "Truth"=6, "Predicted"=6}, {"image"=array28x28[784 elements], "Truth"=6, "Predicted"=6}, {"image"=array28x28[784 elements], "Truth"=5, "Predicted"=5}, {"image"=array28x28[784 elements], "Truth"=9, "Predicted"=9}], [{"image"=array28x28[784 elements], "Truth"=6, "Predicted"=6}, {"image"=array28x28[784 elements], "Truth"=9, "Predicted"=9}, {"image"=array28x28[784 elements], "Truth"=2, "Predicted"=2}, {"image"=array28x28[784 elements], "Truth"=2, "Predicted"=2}, {"image"=array28x28[784 elements], "Truth"=2, "Predicted"=2}, {"image"=array28x28[784 elements], "Truth"=2, "Predicted"=2}, {"image"=array28x28[784 elements], "Truth"=8, "Predicted"=8}, {"image"=array28x28[784 elements], "Truth"=6, "Predicted"=6}, {"image"=array28x28[784 elements], "Truth"=9, "Predicted"=9}, {"image"=array28x28[784 elements], "Truth"=5, "Predicted"=5}], [{"image"=array28x28[784 elements], "Truth"=3, "Predicted"=3}, {"image"=array28x28[784 elements], "Truth"=2, "Predicted"=2}, {"image"=array28x28[784 elements], "Truth"=5, "Predicted"=5}, {"image"=array28x28[784 elements], "Truth"=4, "Predicted"=4}, {"image"=array28x28[784 elements], "Truth"=7, "Predicted"=7}, {"image"=array28x28[784 elements], "Truth"=7, "Predicted"=7}, {"image"=array28x28[784 elements], "Truth"=8, "Predicted"=8}, {"image"=array28x28[784 elements], "Truth"=7, "Predicted"=7}, {"image"=array28x28[784 elements], "Truth"=7, "Predicted"=7}, {"image"=array28x28[784 elements], "Truth"=5, "Predicted"=5}], [{"image"=array28x28[784 elements], "Truth"=2, "Predicted"=2}, {"image"=array28x28[784 elements], "Truth"=7, "Predicted"=7}, {"image"=array28x28[784 elements], "Truth"=7, "Predicted"=7}, {"image"=array28x28[784 elements], "Truth"=8, "Predicted"=8}, {"image"=array28x28[784 elements], "Truth"=0, "Predicted"=0}, {"image"=array28x28[784 elements], "Truth"=6, "Predicted"=6}, {"image"=array28x28[784 elements], "Truth"=7, "Predicted"=7}, {"image"=array28x28[784 elements], "Truth"=2, "Predicted"=2}, {"image"=array28x28[784 elements], "Truth"=0, "Predicted"=0}, {"image"=array28x28[784 elements], "Truth"=0, "Predicted"=0}], [{"image"=array28x28[784 elements], "Truth"=0, "Predicted"=0}, {"image"=array28x28[784 elements], "Truth"=0, "Predicted"=0}, {"image"=array28x28[784 elements], "Truth"=0, "Predicted"=0}, {"image"=array28x28[784 elements], "Truth"=7, "Predicted"=7}, {"image"=array28x28[784 elements], "Truth"=4, "Predicted"=4}, {"image"=array28x28[784 elements], "Truth"=3, "Predicted"=3}, {"image"=array28x28[784 elements], "Truth"=7, "Predicted"=7}, {"image"=array28x28[784 elements], "Truth"=5, "Predicted"=5}, {"image"=array28x28[784 elements], "Truth"=7, "Predicted"=7}, {"image"=array28x28[784 elements], "Truth"=6, "Predicted"=6}], [{"image"=array28x28[784 elements], "Truth"=0, "Predicted"=0}, {"image"=array28x28[784 elements], "Truth"=4, "Predicted"=4}, {"image"=array28x28[784 elements], "Truth"=9, "Predicted"=9}, {"image"=array28x28[784 elements], "Truth"=7, "Predicted"=7}, {"image"=array28x28[784 elements], "Truth"=2, "Predicted"=2}, {"image"=array28x28[784 elements], "Truth"=6, "Predicted"=6}, {"image"=array28x28[784 elements], "Truth"=5, "Predicted"=5}, {"image"=array28x28[784 elements], "Truth"=3, "Predicted"=3}, {"image"=array28x28[784 elements], "Truth"=2, "Predicted"=2}, {"image"=array28x28[784 elements], "Truth"=6, "Predicted"=6}]]
  out "Confusion Matrix":string[][](table)=[["966", "0", "0", "0", "2", "2", "5", "2", "2", "1", "0.986"], ["0", "1115", "2", "4", "0", "3", "2", "1", "8", "0", "0.982"], ["5", "1", "986", "5", "1", "1", "2", "23", "6", "2", "0.955"], ["2", "0", "16", "952", "1", "18", "0", "14", "2", "5", "0.943"], ["1", "1", "5", "0", "915", "0", "7", "4", "3", "46", "0.932"], ["6", "1", "0", "10", "0", "862", "7", "4", "0", "2", "0.966"], ["13", "3", "0", "0", "7", "4", "928", "0", "2", "1", "0.969"], ["2", "9", "13", "5", "0", "0", "0", "990", "1", "8", "0.963"], ["4", "0", "4", "12", "5", "18", "8", "18", "890", "15", "0.914"], ["3", "5", "2", "4", "9", "15", "0", "12", "3", "956", "0.947"], ["0.964", "0.982", "0.959", "0.960", "0.973", "0.934", "0.968", "0.927", "0.971", "0.923", ""]]
  out "Valid_Error":sgl=0.042666666
  out "Valid_Loss":sgl=0.04526825
  in  "Stop_Test":bool
  # "Overview: This example demonstrates the usage of Deep Learning Toolkit for solving hand written digit recognition problem with Convolutional Neural Network (CNN).\nDataset: MNIST http://yann.lecun.com/exdb/mnist/\nRequirements: Deep Learning Toolkit for LabVIEW.\nInstructions:\n1. Download MNIST dataset (4 files) from the link above and extract all files into one directory and provide the path to that directory at \"MNIST Dataset Path\" control.\n2. Set appropriate path at \"Working Dir\" control where the results of the training will be stored.\n3.  Run the VI with current configuration of the training parameters and Learning Rate update policy.\n4. Observe how the training loss is decreasing.\n5. Observe training speed.\n6. Periodically press \"Eval Validation\" button to evaluate Validation Loss/Error.\nNote that validation error evaluation influences the training speed, as the forward network inference is run for whole validation dataset."
  # "7. Hit \"Stop Train\" button when Validation Loss/Errors are not decreasing any more (~10 epochs).\n8. Observe the Test Error value - this represents the final accuracy of the trained network.\n9. Go to the Testing tab.\n10. Draw a digit in Draw Digit Interface and observe correctness of the predictions in the Predictions  indicator. Observe testing speed.\n11. Stop the VI by pressing \"Stop Test\" button on Testing tab.\n12. Go to the Incorrectly Classified Images tab and observe images that were incorrectly predicted by the network from the test dataset.\n13. Navigate to \"Confusion Matrix\" tab and observe the results on Test dataset.\n14. Observe the files generated at \"Working Dir\" directory. Navigate to Working directory. A directory with network name should have been created which should contain 3 files: model configuration file (.cfg), a file with trained weights (.bin), and a network visualization file (.svg) which can be opened in a web browser.\n15. Modify the network by changing network configuration on the block diagram. Go through the steps 3.-12. and observe influence on the test Loss/Error.\n16. (Optional) For deployment please open MNIST_Classifier(Deploy).vi.\n17. (Optional) Change \"NN_Device\" value to \"GPU\" to compare execution speeds on GPU and CPU.\n\nMore Examples:  https://github.com/ngenehub/deepltk_examples"
  # "Displaying images from the dataset that were incorrectly classified by the trained network."
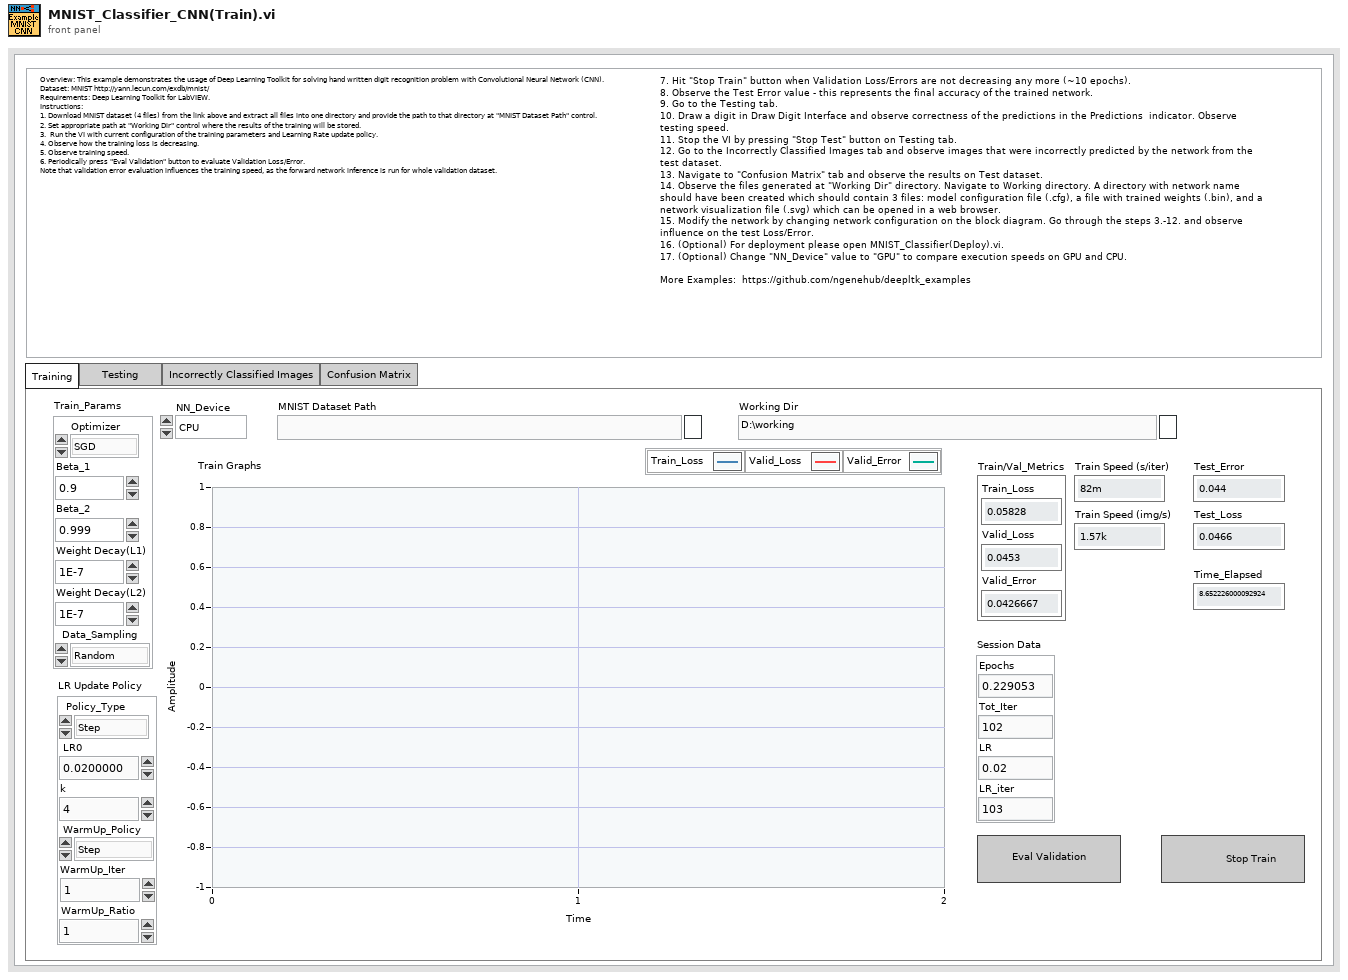
[diagram p1: front panel]
types:
  T1 = enum32{"Training", "Testing           ", "Incorrectly Classified Images", "Confusion Matrix"}
  T2 = cluster{"Filtered x":sgl, "Valid_Loss":sgl, "Valid_Error":sgl}
  T3 = typedef "Deep_Learning_Toolkit_by_Ngene.lvlib/NN_Train_Session_Data.ctl" = cluster{"Epochs":sgl, "Tot_Iter":i32, "LR":sgl, "LR_iter":i32}
  T4 = cluster{"Train_Loss":sgl, "Valid_Loss":sgl, "Valid_Error":sgl}
  T5 = typedef "Deep_Learning_Toolkit_by_Ngene.lvlib/NN_LR_Policy_Cfg.ctl" = cluster{"Policy_Type":T6, "LR0":dbl, "k":sgl, "WarmUp_Policy":enum16{"Step", "Ramp"}, "WarmUp_Iter":i32, "WarmUp_Ratio":sgl}
  T6 = typedef "Deep_Learning_Toolkit_by_Ngene.lvlib/NN_LR_Policy_Type.ctl" = enum16{"Manual", "Step", "Exp", "1/t"}
  T7 = typedef "Deep_Learning_Toolkit_by_Ngene.lvlib/NN_Train_Params.ctl" = cluster{"Optimizer":T8, "Beta_1":sgl, "Beta_2":sgl, "Weight Decay(L1)":sgl, "Weight Decay(L2)":sgl, "Data_Sampling":T9}
  T8 = typedef "Deep_Learning_Toolkit_by_Ngene.lvlib/NN_Train_Optimizer.ctl" = enum16{"SGD", "Adam", "Adagrad", "Adadelta", "RMSProp", "Nesterov"}
  T9 = typedef "Deep_Learning_Toolkit_by_Ngene.lvlib/NN_Train_Data_Sampling.ctl" = enum16{"Random", "Sequential"}
  T10 = typedef "Deep_Learning_Toolkit_by_Ngene.lvlib/NN_Device.ctl" = enum16{"CPU", "GPU"}
  T11 = cluster{"Width":u16, "Style":enum32{"Solid", "Dash", "Dot", "DashDot", "DashDotDot"}}
  T12 = typedef "Img_GrayScale.ctl" = cluster{"image":sgl[][], "Truth":i32, "Predicted":i32}
  T13 = typedef "Deep_Learning_Toolkit_by_Ngene.lvlib/NN_Layer_Config(Conv2D).ctl" = cluster{"Name":string, "Conv_Params":T14, "BN?":bool, "BN_Params":T16, "Activation":T17, "Has Bias?":bool, "Init_Params":T18, "Custom_Params":string}
  T14 = typedef "Deep_Learning_Toolkit_by_Ngene.lvlib/NN_Layer_Params(Conv2D).ctl" = cluster{"Filters":i32, "Kernel_Size":i32, "Stride":i32, "Pad_Type":T15, "Pad_Size":i32}
  T15 = typedef "Deep_Learning_Toolkit_by_Ngene.lvlib/NN_Conv2D_Padding_Type.ctl" = enum16{"Pad_Size", "Valid", "Same"}
  T16 = typedef "Deep_Learning_Toolkit_by_Ngene.lvlib/NN_BN_Params.ctl" = cluster{"epsilon":sgl, "momentum":sgl}
  T17 = typedef "Deep_Learning_Toolkit_by_Ngene.lvlib/NN_Activation_Type.ctl" = enum16{"Sigmoid", "ReLU", "LReLU", "ReLU6", "tanh", "Swish", "Mish", "None"}
  T18 = typedef "Deep_Learning_Toolkit_by_Ngene.lvlib/NN_Layer_Init_Params.ctl" = cluster{"Init_Type":T19, "Value":sgl}
  T19 = typedef "Deep_Learning_Toolkit_by_Ngene.lvlib/NN_Layer_Weight_Init_Type.ctl" = enum16{"Const", "Uniform", "Gaussian", "Xavier"}
  T20 = typedef "Deep_Learning_Toolkit_by_Ngene.lvlib/NN_Layer_Config(FC).ctl" = cluster{"Name":string, "Size":i32, "BN":bool, "BN_Params":T16, "Activation":T17, "Has Bias?":bool, "Init_Params":T18, "Custom_Params":string}
  T21 = typedef "Deep_Learning_Toolkit_by_Ngene.lvlib/NN_Save_Before_Destroy_Options.ctl" = cluster{"CFG?":bool, "Weights?":bool, "Render?":bool}
  T22 = typedef "Deep_Learning_Toolkit_by_Ngene.lvlib/NN_Layer_Config(Input3D).ctl" = cluster{"Name":string, "Dims":T23, "Data_Type":T24, "Shifts":sgl[], "Scales":sgl[]}
  T23 = typedef "Deep_Learning_Toolkit_by_Ngene.lvlib/NN_Dims(C,H,W).ctl" = cluster{"C":i32, "H":i32, "W":i32}
  T24 = typedef "Deep_Learning_Toolkit_by_Ngene.lvlib/NN_Data_type.ctl" = enum16{"I8", "U8", "I16", "U16", "U32 ARGB", "SGL"}
  T25 = typedef "Deep_Learning_Toolkit_by_Ngene.lvlib/NN_DataSets_All(In3D_Out1D).ctl" = cluster{"Train":T26, "Validation":T26, "Test":T26}
  T26 = typedef "Deep_Learning_Toolkit_by_Ngene.lvlib/NN_DataSet(In3D_Out1D).ctl" = cluster{"Inputs Ref.":variant, "Outputs Ref.":T27, "Dataset_Size":i32, "Dims_In":T23, "Dims_Out":i32, "Labels":string[], "File Paths":path[]}
  T27 = typedef "Deep_Learning_Toolkit_by_Ngene.lvlib/NN_Data_ref(2D_SGL).ctl" = refnum<data-value>
  T28 = typedef "Deep_Learning_Toolkit_by_Ngene.lvlib/NN.ctl" = cluster{"Name":string, "No of Layers":i32, "mBatch":i32, "Layers":T29[], "Dimty":T30, "Dims_In":T23, "Dims_Out":T23, "Working_Dir":path, "Train?":bool, "Train_Params":T7, "LR_Update_Policy":T5, "Session Data":T3, "Ground_truth":T31, "NNg_hdls":T32, "NN_Device":T10, "GPU Id":i32, "Labels":string[], "Receptive Field":T33[], "Loss_Type":T34, "Loss_Cfg_Prms":variant, "NNG_WS":T35}
  T29 = typedef "Deep_Learning_Toolkit_by_Ngene.lvlib/NN_Layer_ref.ctl" = refnum<data-value>
  T30 = typedef "Deep_Learning_Toolkit_by_Ngene.lvlib/NN_In_Out_Dim-ty.ctl" = enum8{"In1D_Out1D", "In3D_Out1D", "In3D_Out3D", "In3D_OutBBox"}
  T31 = typedef "Deep_Learning_Toolkit_by_Ngene.lvlib/NN_Ground_truth.ctl" = cluster{"Y":variant}
  T32 = typedef "Deep_Learning_Toolkit_by_Ngene.lvlib/nng_cuda_handles.ctl" = cluster{"cudnn":u64, "cublas":u64, "stream":u64, "curand":u64}
  T33 = typedef "Deep_Learning_Toolkit_by_Ngene.lvlib/NN_Dims(V,H).ctl" = cluster{"V":i32, "H":i32}
  T34 = typedef "Deep_Learning_Toolkit_by_Ngene.lvlib/NN_Loss_Type.ctl" = enum16{"None", "MSE", "CrossEntropy", "YOLO_v2", "YOLO_v4"}
  T35 = typedef "Deep_Learning_Toolkit_by_Ngene.lvlib/NNG_WS.ctl" = cluster{"NNG_WS_Mem":T36, "Max_WS_Size":i64}
  T36 = typedef "Deep_Learning_Toolkit_by_Ngene.lvlib/NNg_WS_Mem_DVR.ctl" = refnum<data-value>
  T37 = typedef "Deep_Learning_Toolkit_by_Ngene.lvlib/NN_Eval_Params.ctl" = cluster{"Loss":sgl, "Error":sgl}
  T38 = typedef "Deep_Learning_Toolkit_by_Ngene.lvlib/NN_Layer.ctl" = cluster{"Name":string, "Layer_Data":variant, "Layer_Type":T39, "Dims_In":T23, "Layers_In":variant, "Dims_Out":T23, "Layers_Out":variant, "Metrics":T40, "GPU_Data":variant, "mBatch":i32, "NN_Device":T10, "NNg_hdls":T32, "Train?":bool, "Dimty":T41, "RecptField":T42}
  T39 = typedef "Deep_Learning_Toolkit_by_Ngene.lvlib/NN_Layer_Type.ctl" = enum16{"Input1D", "Input3D", "Conv1D", "Conv2D", "Conv2D_Adv", "MaxPool", "AvgPool", "UpSample", "DropOut3D", "ShortCut", "Concat", "SoftMax3D", "FC", "DropOut", "Softmax", "Flatten", "YOLO_v2", "YOLO_v4", "Activation", "BatchNormalization", "Unsupported"}
  T40 = typedef "Deep_Learning_Toolkit_by_Ngene.lvlib/NN_Layer_Metrics.ctl" = cluster{"Data":dbl, "Params":dbl, "Ops":dbl}
  T41 = typedef "Deep_Learning_Toolkit_by_Ngene.lvlib/NN_Layer_Dimty.ctl" = enum16{"1D", "3D"}
  T42 = typedef "Deep_Learning_Toolkit_by_Ngene.lvlib/NN_Layer_RF_State.ctl" = cluster{"Dims":T33, "J":T33}
  T43 = cluster{"left":i16, "top":i16, "right":i16, "bottom":i16}
  T44 = typedef "LVMouseTypeDef.ctl" = cluster{"Mouse Position":cluster{"X":i32, "Y":i32}, "Mouse Modifiers":cluster{"Button Down":bool, "Shift Mod":bool, "Menu Mod":bool, "Option Mod":bool}}
  T45 = typedef "imagedata.ctl" = cluster{"image type":i32, "image depth":i32, "image":u8[], "mask":u8[], "colors":u32[], "Rectangle":cluster{"left":i16, "top":i16, "right":i16, "bottom":i16}}
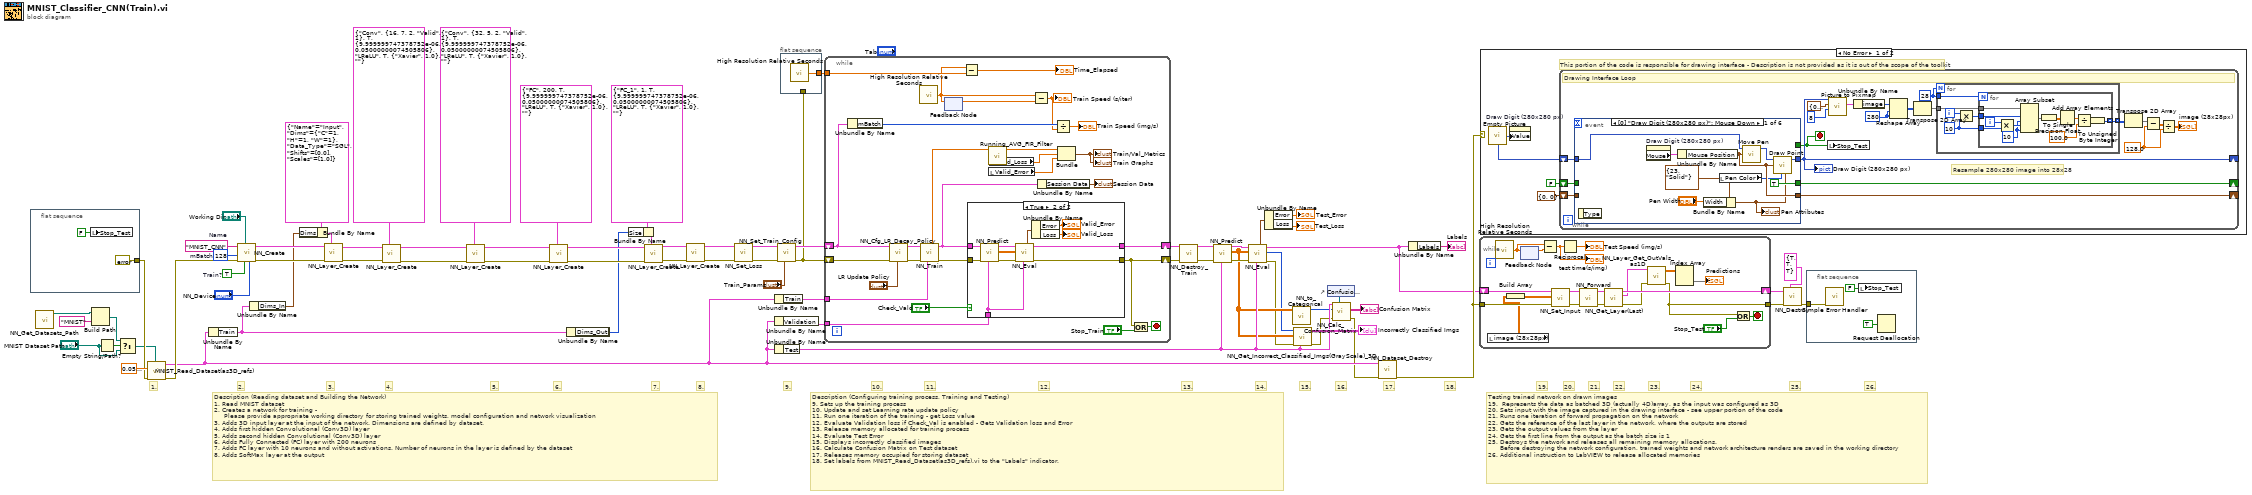
[diagram p0: block diagram]
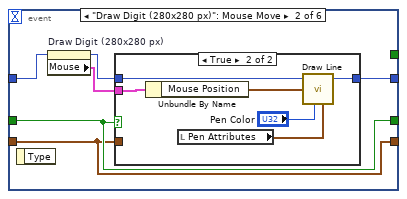
[diagram p3: hidden frame]
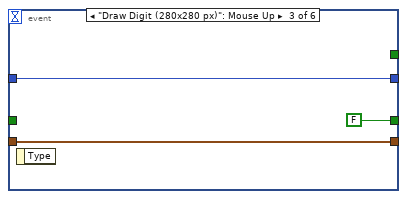
[diagram p5: hidden frame]
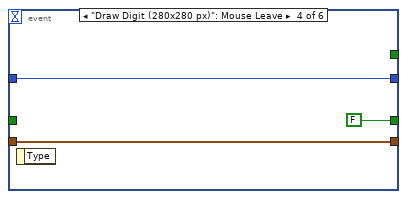
[diagram p6: hidden frame]
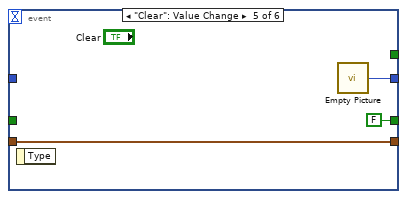
[diagram p7: hidden frame]
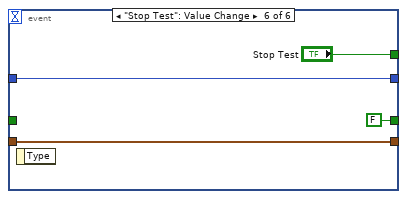
[diagram p8: hidden frame]
diagram:
  w52 = TRUE  # Train?
  w64 = 128  # mBatch
  w72 = "MNIST_CNN"  # Name
  # "18."
  # "16."
  # "26."
  # "25."
  # "Testing trained network on drawn images \n19.  Represents the data as batched 3D (actually 4D)array, as the input was configured as 3D\n20. Sets input with the image captured in the drawing interface - see upper portion of the code\n21. Runs one iteration of forward propagation on the network\n22. Gets the reference of the last layer in the network, where the outputs are stored\n23. Gets the output values from the layer\n24. Gets the first line from the output as the batch size is 1\n25. Destroys the network and releases all remaining memory allocations.\n      Before destroying the network configuration, trained weights and network architecture renders are saved in the working directory\n26. Additional instruction to LabVIEW to release allocated memories"
  # "24."
  # "Description (Configuring training process, Training and Testing)\n9. Sets up the training process\n10. Update and set Learning rate update policy\n11. Run one iteration of the training - get Loss value\n12. Evaluate Validation loss if Check_Val is enabled - Gets Validation loss and Error\n13. Release memory allocated for training process\n14. Evaluate Test Error\n15. Displays incorrectly classified images\n16. Calculate Confusion Matrix on Test dataset  \n17. Releases memory occupied for storing dataset\n18. Set labels from MNIST_Read_Dataset(as3D_refs).vi to the \"Labels\" indicator."
  # "Description (Reading dataset and Building the Network)\n1. Read MNIST dataset\n2. Creates a network for training - \n     Please provide appropriate working directory for storing trained weights, model configuration and network visualization\n3. Adds 3D input layer at the input of the network. Dimensions are defined by dataset.\n4. Adds first hidden Convolutional (Conv3D) layer \n5. Adds second hidden Convolutional (Conv3D) layer\n6. Adds Fully Connected (FC) layer with 200 neurons\n7. Adds FC layer with 10 neurons and without activations. Number of neurons in the layer is defined by the dataset\n8. Adds SoftMax layer at the output"
  # "23."
  # "22."
  # "21."
  # "20."
  # "19."
  # "17."
  # "15."
  # "14."
  # "13."
  # "12."
  # "11."
  # "10."
  # "9."
  # "8."
  # "7."
  # "6."
  # "5."
  # "4."
  # "3."
  # "2."
  # "1."
  n1 = flat-sequence {
    tunnel: [errorcluster {"status"=FALSE, "code"=0, "source"=""} ("error in (no error)")] -> w56
    frame #0 {
      n2 = local write "Stop_Test"(FALSE ("Stop_Test")) -> ()
    }
  }
  n3 = call "NN_Get_Datasets_Path.vi"() -> ("Datasets path"=w5:path)  [unwired: 11 in]
  n4 = Build Path(base path=w5, name or relative path="MNIST") -> (appended path=w9:path)
  n5 = Empty String/Path?(string/path="MNIST Dataset Path") -> (empty?=w8:bool)
  n6 = Select(t=w9, s=w8, f="MNIST Dataset Path") -> (s? t:f=w6:path)
  n7 = call "MNIST_Read_Dataset(as3D_refs).vi"("MNIST Dataset Path"=w6, "error in"=w56, "Validation_Size"=sgl 0.05 ("Valid_data_Size")) -> ("error out"=w73:errorcluster, "Data(3D)_Refs"=w34:T25)  [unwired: 7 in]
  n8 = Unbundle By Name(w34) -> ("Train"=w33:T26)
  n9 = call <vilib>:"NN_Create.vi"("NN_Device"="NN_Device", "Train? (false)"=w52, "Working Dir"="Working Dir", "error in (no error)"=w73, "mBatch (1)"=w64, "Name"=w72) -> ("error out"=w70:errorcluster, "NN out"=w71:T28)  [unwired: 4 in]
  n10 = Unbundle By Name(w33) -> ("Dims_In"=w35:T23)
  n11 = Bundle By Name(cluster=T22 {"Name"="Input", "Dims"={"C"=1, "H"=1, "W"=1}, "Data_Type"=enum."SGL", "Shifts"=[0.0], "Scales"=[1.0]} ("Cluster"), "Dims"=w35) -> (w57:T22)
  n12 = call-poly <vilib>:"NN_Layer_Create.vi"("Input3D_Cfg"=w57, "error in (no error)"=w70, "NN In"=w71) -> ("error out"=w45:errorcluster, "NN out"=w21:T28)  [unwired: 6 in, 1 out]
  n13 = call-poly <vilib>:"NN_Layer_Create.vi"("Conv2D_Cfg"=T13 {"Name"="Conv", "Conv_Params"={"Filters"=16, "Kernel_Size"=7, "Stride"=2, "Pad_Type"=enum."Valid", "Pad_Size"=1}, "BN?"=TRUE, "BN_Params"={"epsilon"=1e-05, "momentum"=0.05}, "Activation"=enum."LReLU", "Has Bias?"=TRUE, "Init_Params"={"Init_Type"=enum."Xavier", "Value"=1.0}, "Custom_Params"=""} ("Layer_Config_Params"), "error in (no error)"=w45, "NN in"=w21) -> ("error out"=w42:errorcluster, "NN out"=w19:T28)  [unwired: 6 in, 1 out]
  n14 = call-poly <vilib>:"NN_Layer_Create.vi"("Conv2D_Cfg"=T13 {"Name"="Conv", "Conv_Params"={"Filters"=32, "Kernel_Size"=5, "Stride"=2, "Pad_Type"=enum."Valid", "Pad_Size"=1}, "BN?"=TRUE, "BN_Params"={"epsilon"=1e-05, "momentum"=0.05}, "Activation"=enum."LReLU", "Has Bias?"=TRUE, "Init_Params"={"Init_Type"=enum."Xavier", "Value"=1.0}, "Custom_Params"=""} ("Layer_Config_Params"), "error in (no error)"=w42, "NN in"=w19) -> ("error out"=w40:errorcluster, "NN out"=w43:T28)  [unwired: 6 in, 1 out]
  n15 = call-poly <vilib>:"NN_Layer_Create.vi"("FC_Cfg"=T20 {"Name"="FC", "Size"=200, "BN"=TRUE, "BN_Params"={"epsilon"=1e-05, "momentum"=0.05}, "Activation"=enum."LReLU", "Has Bias?"=TRUE, "Init_Params"={"Init_Type"=enum."Xavier", "Value"=1.0}, "Custom_Params"=""} ("Layer_Config_Params"), "error in (no error)"=w40, "NN in"=w43) -> ("error out"=w47:errorcluster, "NN out"=w46:T28)  [unwired: 6 in, 1 out]
  n16 = Unbundle By Name(w33) -> ("Dims_Out"=w32:i32)
  n17 = Bundle By Name(cluster=T20 {"Name"="FC_1", "Size"=1, "BN"=TRUE, "BN_Params"={"epsilon"=1e-05, "momentum"=0.05}, "Activation"=enum."LReLU", "Has Bias?"=TRUE, "Init_Params"={"Init_Type"=enum."Xavier", "Value"=1.0}, "Custom_Params"=""} ("Layer_Config_Params"), "Size"=w32) -> (w44:T20)
  n18 = call-poly <vilib>:"NN_Layer_Create.vi"("FC_Cfg"=w44, "error in (no error)"=w47, "NN in"=w46) -> ("error out"=w60:errorcluster, "NN out"=w61:T28)  [unwired: 6 in, 1 out]
  n19 = call-poly <vilib>:"NN_Layer_Create.vi"("error in (no error)"=w60, "NN in"=w61) -> ("error out"=w38:errorcluster, "NN out"=w41:T28)  [unwired: 7 in, 1 out]
  n20 = call-poly <vilib>:"NN_Set_Loss.vi"("error in (no error)"=w38, "NN in"=w41) -> ("error out"=w37:errorcluster, "NN out"=w39:T28)  [unwired: 8 in]
  n21 = Unbundle By Name(w34) -> ("Train"=w36:T26)
  n22 = Unbundle By Name(w34) -> ("Validation"=w63:T26)
  n23 = Unbundle By Name(w34) -> ("Test"=w23:T26)
  n24 = call <vilib>:"NN_Set_Train_Config.vi"("NN_Train_Params"="Train_Params", "error in (no error)"=w37, "NN in"=w39) -> ("error out"=w53:errorcluster, "NN out"=w54:T28)  [unwired: 7 in]
  n25 = flat-sequence {
    tunnel: [w76] -> w66
    tunnel: w53 -> [_]
    frame #0 {
      n26 = call <vilib>:"High Resolution Relative Seconds.vi"() -> ("relative seconds"=w76:dbl)
    }
  }
  n27 = while {
    shift-right: [w84] -> w28
    shift-left: w53 -> [w78]
    shift-right: [w81] -> w29
    shift-left: w54 -> [w79]
    tunnel: w66 -> [w93]
    tunnel: w36 -> [w83]
    tunnel: w63 -> [w77]
    stop <- w101 stop-if-true
    n28 = Unbundle By Name(w79) -> ("mBatch"=w89:i32)
    n29 = call <vilib>:"NN_Cfg_LR_Decay_Policy.vi"("LR_Decay_Params"="LR Update Policy", "error in (no error)"=w78, "NN in"=w79) -> ("error out"=w96:errorcluster, "NN out"=w102:T28)  [unwired: 7 in]
    n30 = call <vilib>:"High Resolution Relative Seconds.vi"() -> ("relative seconds"=w92:dbl)
    n31 = call <vilib>:"NN_Train.vi"("Train Dataset"=w83, "error in (no error)"=w96, "NN in"=w102) -> ("error out"=w85:errorcluster, "NN out"=w80:T28, "Loss"=w97:sgl)  [unwired: 3 in, 3 out]
    n32 = feedback #1() -> (w103:dbl)  [unwired: 1 in]
    n33 = feedback-in #1(w92) -> ()
    n34 = Subtract(x=w92, y=w93) -> (x-y=→"Time_Elapsed":dbl)
    n35 = case shown="True" "Check_Vald" {
      tunnel: w80 -> [w104 w116]
      tunnel: w85 -> [w105 w112]
      tunnel: [w105 w114] -> w84
      tunnel: [w104 w115] -> w81
      tunnel: w77 -> [_ w109]
      frame False {
      }
      frame True {
        n36 = call-poly <vilib>:"NN_Predict.vi"("Dataset"=w109, "error in (no error)"=w112, "NN in"=w116) -> ("error out"=w111:errorcluster, "Predictions"=w110:sgl[][], "NN out"=w113:T28)  [unwired: 6 in]
        n37 = call-poly <vilib>:"NN_Eval.vi"("Dataset"=w109, "error in (no error)"=w111, "Predictions"=w110, "NN in"=w113) -> ("error out"=w114:errorcluster, "NN out"=w115:T28, "NN_Eval_Params"=w108:T37)  [unwired: 4 in, 1 out]
        n38 = Unbundle By Name(w108) -> ("Error"=→"Valid_Error":sgl, "Loss"=→"Valid_Loss":sgl)
      }
    }
    n39 = call <vilib>:"Running_AVG_FIR_Filter.vi"("Numeric"=w97) -> ("Filtered x"=w98:sgl)  [unwired: 10 in]
    n40 = local read "Valid_Error"() -> (w95:sgl)
    n41 = local read "Valid_Loss"() -> (w100:sgl)
    n42 = Subtract(x=w92, y=w103) -> (x-y=w87:dbl)
    "Train Speed (s/iter)" <- w87
    n43 = Unbundle By Name(w80) -> ("Session Data"=→"Session Data":T3)
    n44 = Divide(x=w89, y=w87) -> (x/y=→"Train Speed (img/s)":dbl)
    n45 = Bundle("Filtered x"=w98, "Valid_Loss"=w100, "Valid_Error"=w95) -> (→"Train Graphs" →"Train/Val_Metrics":T2)  [unwired: 1 in]
    n46 = Compound Arithmetic op=OR(w84, "Stop_Train") -> (w101:bool)
  }
  n47 = call <vilib>:"NN_Destroy_Train.vi"("error in (no error)"=w28, "NN in"=w29) -> ("error out"=w25:errorcluster, "NN out"=w27:T28)  [unwired: 8 in]
  n48 = call-poly <vilib>:"NN_Predict.vi"("Dataset"=w23, "error in (no error)"=w25, "NN in"=w27) -> ("error out"=w24:errorcluster, "Predictions"=w17:sgl[][], "NN out"=w26:T28)  [unwired: 6 in]
  n49 = call-poly <vilib>:"NN_Eval.vi"("Dataset"=w23, "error in (no error)"=w24, "Predictions"=w17, "NN in"=w26) -> ("error out"=w14:errorcluster, "Incrct_Class_idx"=w4:i32[], "NN out"=w16:T28, "NN_Eval_Params"=w1:T37)  [unwired: 4 in]
  n50 = Unbundle By Name(w1) -> ("Error"=→"Test_Error":sgl, "Loss"=→"Test_Loss":sgl)
  n51 = call <vilib>:"NN_to_Categorical.vi"("Prediction"=w17) -> ("Label_Idx"=w18:i32[])  [unwired: 10 in]
  n52 = call "NN_Get_Incorrect_Classified_Imgs(GrayScale)_3D.vi"("Test_Data"=w23, "error in (no error)"=w14, "Predictions"=w17, "MisClassed_idx"=w4) -> ("error out"=w13:errorcluster, "Images(GrayScale)"=→"Incorrectly Classified Imgs":T12[][])  [unwired: 6 in]
  n53 = control-ref of="Confusion Matrix"() -> (w30:refnum<vi>)
  n54 = call-poly <vilib>:"NN_Calc_Confusion_Matrix.vi"("Confusion Matrix (Table) ref."=w30, "error in (no error)"=w13, "Predictions"=w18, "Dataset"=w23) -> ("error out"=w12:errorcluster, "Confusion Matrix (Table)"=→"Confusion Matrix":string[][])  [unwired: 3 in, 3 out]
  n55 = call-poly <vilib>:"NN_Dataset_Destroy.vi"("error in (no error)"=w12, "Datasets_All(In3D_Out1D)"=w34) -> ("error out"=w55:errorcluster)  [unwired: 9 in]
  n56 = Unbundle By Name(w16) -> ("Labels"=→"Labels":string[])
  n57 = while {
    shift-right: [w135] -> w68
    shift-left: w16 -> [w128]
    tunnel: w55 -> [w126]
    tunnel: [w118] -> w67
    stop <- w133 stop-if-true
    n58 = local read "image (28x28px)"() -> (w124:sgl[][])
    n59 = call <vilib>:"High Resolution Relative Seconds.vi"() -> ("relative seconds"=w131:dbl)
    n60 = Build Array(w124) -> (w117:sgl[][][])
    n61 = feedback #2() -> (w132:dbl)  [unwired: 1 in]
    n62 = feedback-in #2(w131) -> ()
    n63 = Subtract(x=w131, y=w132) -> (x-y=w130:dbl)
    "test time(s/img)" <- w130
    n64 = call-poly <vilib>:"NN_Set_Input.vi"("error in (no error)"=w126, "Data_In(3D_SGL)"=w117, "NN in"=w128) -> ("error out"=w125:errorcluster, "NN out"=w127:T28)  [unwired: 7 in]
    n65 = Reciprocal(x=w130) -> (1/x=→"Test Speed (img/s)":dbl)
    n66 = call <vilib>:"NN_Forward.vi"("error in (no error)"=w125, "NN in"=w127) -> ("error out"=w134:errorcluster, "NN out"=w136:T28)  [unwired: 6 in, 2 out]
    n67 = call <vilib>:"NN_Get_Layer(Last).vi"("error in (no error)"=w134, "NN in"=w136) -> ("error out"=w119:errorcluster, "Last_Layer"=w123:T38, "NN out"=w135:T28)  [unwired: 6 in, 1 out]
    n68 = call <vilib>:"NN_Layer_Get_OutVals_as1D.vi"("error in (no error)"=w119, "Layer"=w123) -> ("error out"=w118:errorcluster, "Out(as1D)"=w122:sgl[][])  [unwired: 8 in]
    n69 = Index Array(array=w122) -> (element=→"Predictions":sgl[])  [unwired: 2 in]
    n70 = Or(x=w118, y="Stop_Test") -> (x .or. y?=w133:bool)
  }
  n71 = case shown="No Error" w55 {
    frame No Error {
      # "This portion of the code is responsible for drawing interface - Description is not provided as it is out of the scope of the toolkit"
      n72 = call "Empty Picture"() -> ("empty picture"=w139:picture)
      n73 = property on="Draw Digit (280x280 px)" class="Pict"("Value"=w139) -> ()  [unwired: 2 in, 2 out]
      n74 = while {
        shift-right: [w154] -> _
        shift-left: w139 -> [w159]
        shift-right: [w157] -> _
        shift-left: FALSE -> [w158]
        shift-right: [w155] -> _
        shift-left: cluster{"X":i32, "Y":i32} {"X"=0, "Y"=0} ("Mouse Position") -> [w156]
        stop <- w144 stop-if-true
        w141 = sgl 128.0 ("dimension size")
        w145 = 280 ("dimension size")
        w147 = 28
        # "Resample 280x280 image into 28x28"
        # "Drawing Interface Loop"
        n75 = event shown="[0] \"Draw Digit (280x280 px)\": Mouse Down" {
          selector: _ -> [_ _ _ _ _ _]
          dyn-events: _ -> [_ _ _ _ _ _]
          timeout: _ -> [_ _ _ _ _ _]
          tunnel: [_ _ _ _ _ "Stop Test"] -> w144
          tunnel: [w184 w191 w202 w205 w208 w211] -> w154
          tunnel: w159 -> [w186 w190 w202 w205 _ w211]
          tunnel: w158 -> [_ w189 _ _ _ _]
          tunnel: [TRUE w189 FALSE FALSE FALSE FALSE] -> w157
          tunnel: w156 -> [_ w188 w200 w204 w207 w210]
          tunnel: [w182 w188 w200 w204 w207 w210] -> w155
          event "Draw Digit (280x280 px)": Mouse Down {
            # "Set the pen position, and draw an initial point or line."
            n76 = event-data() -> ()  [unwired: 1 in, 1 out]
            n77 = property on="Draw Digit (280x280 px)" class="Pict"() -> ("Mouse"=w187:T44)  [unwired: 2 in, 2 out]
            n78 = Unbundle By Name(w187) -> ("Mouse Position"=w182:cluster{"X":i32, "Y":i32})
            n79 = Bundle By Name(cluster=T11 {"Width"=23, "Style"=enum."Solid"} ("Pen Attributes"), "Width"="Pen Width") -> (w178:T11)
            "Pen Attributes" <- w178
            n80 = local read "Pen Color"() -> (w181:u32)
            n81 = call <vilib>:"Move Pen.vi"("new position"=w182, "picture"=w186) -> ("new picture"=w185:picture)  [unwired: 3 in]
            n82 = call <vilib>:"Draw Point.vi"("picture"=w185, "point(x,y)"=w182, "color(black)"=w181, "pen"=w178) -> ("new picture"=w184:picture)  [unwired: 5 in]
          }
          event "Draw Digit (280x280 px)": Mouse Move {
            # "Only draw if a Mouse Down event has occurred, but not a Mouse Up. Then, determine if the user is Drawing a point, a line, or selecting a subset and perform those operations in the case structure."
            n83 = event-data() -> ()  [unwired: 1 in, 1 out]
            n84 = property on="Draw Digit (280x280 px)" class="Pict"() -> ("Mouse"=w192:T44)  [unwired: 2 in, 2 out]
            n85 = case shown="True" w189 {
              tunnel: w190 -> [w193 w199]
              tunnel: w192 -> [_ w198]
              tunnel: [w193 w196] -> w191
              tunnel: w188 -> [_ _]
              frame False {
              }
              frame True {
                n86 = Unbundle By Name(w198) -> ("Mouse Position"=w197:cluster{"X":i32, "Y":i32})
                n87 = local read "Pen Attributes"() -> (w195:T11)
                n88 = call <vilib>:"Draw Line.vi"("picture"=w199, "end point"=w197, "color(black)"="Pen Color", "pen"=w195) -> ("new picture"=w196:picture)  [unwired: 5 in]
              }
            }
          }
          event "Draw Digit (280x280 px)": Mouse Up {
            # "When the user is finished drawing, we complete the operation. The only operation that we need to complete the Select Subset operation."
            n89 = event-data() -> ()  [unwired: 1 in, 1 out]
          }
          event "Draw Digit (280x280 px)": Mouse Leave {
            # "Change to the default cursor when the mouse leaves the picture."
            n90 = event-data() -> ()  [unwired: 1 in, 1 out]
          }
          event "Clear": Value Change {
            # "Erase the picture."
            n91 = event-data() -> ()  [unwired: 1 in, 1 out]
            n92 = call "Empty Picture"() -> ("empty picture"=w208:picture)
          }
          event "Stop Test": Value Change {
            # "Stop the VI."
            n93 = event-data() -> ()  [unwired: 1 in, 1 out]
          }
        }
        "Draw Digit (280x280 px)" <- w154
        n94 = local write "Stop_Test"(w144) -> ()
        n95 = call <vilib>:"Picture to Pixmap.vi"("depth"=8, "rect"=T43 {"left"=0, "top"=0, "right"=280, "bottom"=280}, "picture"=w154) -> ("image data"=w152:T45)  [unwired: 7 in, 1 out]
        n96 = Unbundle By Name(w152) -> ("image"=w150:u8[])
        n97 = Reshape Array(w150, w145, w145) -> (w149:u8[][])
        n98 = Transpose 2D Array(2D array=w149) -> (transposed array=w148:u8[][])
        n99 = for {
          N: w147 -> [_]
          tunnel: w148 -> [w165]
          tunnel: w147 -> [w164]
          tunnel: [w160] -> w146 mode=indexing
          i -> [w163]
          w161 = 10 ("x")
          n100 = Multiply(x=w163, y=w161) -> (x*y=w162:i32)
          n101 = for {
            N: w164 -> [_]
            tunnel: w165 -> [w177]
            tunnel: w162 -> [w176]
            tunnel: w161 -> [w173]
            tunnel: [w166] -> w160 mode=indexing
            i -> [w175]
            w172 = 10 ("length")
            n102 = Multiply(x=w175, y=w173) -> (x*y=w174:i32)
            n103 = Array Subset(array=w177, index (row)=w176, length (row)=w172, index (col)=w174, length (col)=w172) -> (w171:u8[][])
            n104 = To Single Precision Float(number=w171) -> (single precision float=w170:sgl[][])
            n105 = Add Array Elements(numeric array=w170) -> (sum=w169:sgl)
            n106 = Divide(x=w169, y=sgl 100.0 ("x")) -> (x/y=w167:sgl)
            n107 = To Unsigned Byte Integer(number=w167) -> (unsigned 8bit integer=w166:u8)
          }
        }
        n108 = Transpose 2D Array(2D array=w146) -> (transposed array=w142:u8[][])
        n109 = Subtract(x=w142, y=w141) -> (x-y=w143:sgl[][])
        n110 = Divide(x=w143, y=w141) -> (x/y=→"image (28x28px)":sgl[][])
      }
    }
    frame Error {
    }
  }
  n111 = call <vilib>:"NN_Destroy.vi"("Save (T, T, T)"=T21 {"CFG?"=TRUE, "Weights?"=TRUE, "Render?"=TRUE} ("Save_Config"), "error in (no error)"=w67, "NN in"=w68) -> ("error out"=w69:errorcluster)  [unwired: 7 in, 1 out]
  n112 = flat-sequence {
    tunnel: w69 -> [w214]
    frame #0 {
      n113 = call <vilib>:"Simple Error Handler.vi"("error in (no error)"=w214) -> ()  [unwired: 4 in, 5 out]
      n114 = local write "Stop_Test"(FALSE ("Stop_Test")) -> ()
      n115 = Request Deallocation(TRUE ("flag")) -> ()
    }
  }
